vi "a_3__b_3_SUB.vi"(1 "b":dbl, 2 "a":dbl) -> (0 "a^3+b^3":dbl)   [LabVIEW 2026]
panel:
  # "1. Create a vi to perform the operation a3+b3, using this vi as subvi perform (a+b)3"
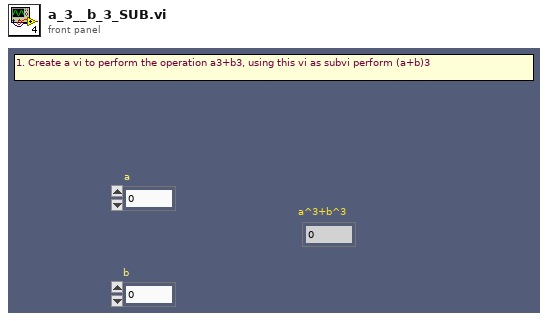
[diagram p1: front panel]
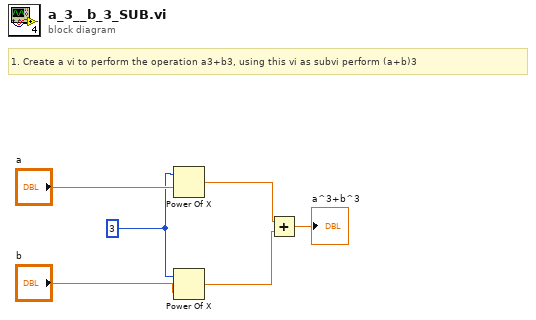
[diagram p0: block diagram]
diagram:
  w5 = 3
  # "1. Create a vi to perform the operation a3+b3, using this vi as subvi perform (a+b)3"
  n1 = Power Of X(1:"a", 2:w5) -> (0:w3:dbl)
  n2 = Power Of X(1:"b", 2:w5) -> (0:w2:dbl)
  n3 = Add(x=w3, y=w2) -> (x+y=→"a^3+b^3":dbl)
